vi "SelectFitRange (SubVI).vi"(7 "Fit type":T1, 9 "delta y values":dbl[](array[numeric]), 10 "y values":dbl[](array[numeric]), 11 "x values":dbl[](array[numeric])) -> (1 "Selected delta y values":dbl[](array[numeric]), 2 "Selected y values":dbl[](array[numeric]), 3 "Selected x values":dbl[](array[numeric]))   [LabVIEW 2016]
uses:
  Utils/Enum_TypeDefinitions/Enum_TypeDef_ParabolaFitType.ctl
panel:
  out "Index of extreme":i32
  out "Righthand side":i32
  out "Lefthand side":i32
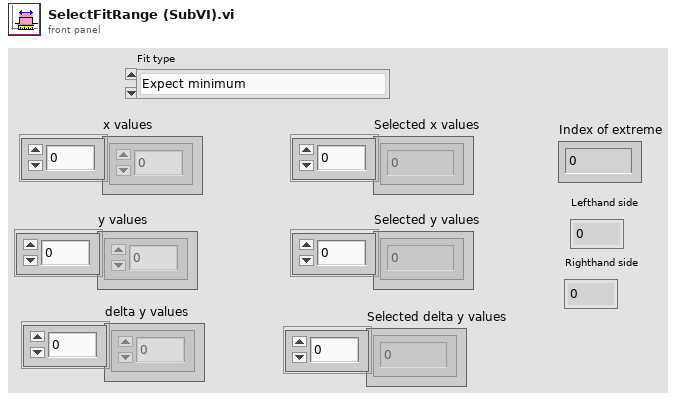
[diagram p1: front panel]
types:
  T1 = typedef "Enum_TypeDef_ParabolaFitType.ctl" = enum16{"Expect minimum", "Expect maximum"}
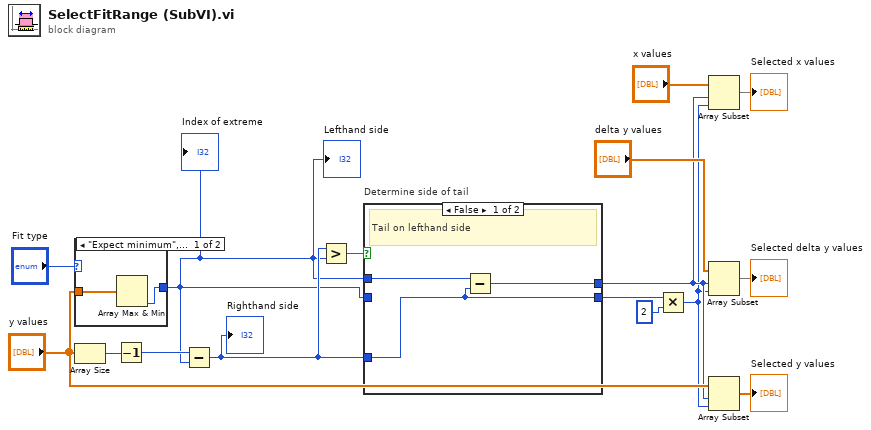
[diagram p0: block diagram]
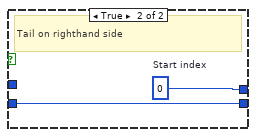
[diagram p2: hidden frame]
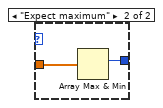
[diagram p3: hidden frame]
diagram:
  n1 = case shown="\"Expect minimum\", Default" "Fit type" {
    tunnel: [w17 w20] -> w5
    tunnel: "y values" -> [w18 w19]
    frame "Expect minimum", Default {
      n2 = Array Max & Min(array=w18) -> (min index (indices)=w17:i32)  [unwired: 3 out]
    }
    frame "Expect maximum" {
      n3 = Array Max & Min(array=w19) -> (max index (indices)=w20:i32)  [unwired: 3 out]
    }
  }
  "Lefthand side" <- w5
  "Index of extreme" <- w5
  n4 = Array Size(array="y values") -> (size(s)=w10:i32)
  n5 = Decrement(x=w10) -> (x-1=w11:i32)
  n6 = Subtract(x=w11, y=w5) -> (x-y=w6:i32)
  "Righthand side" <- w6
  n7 = Greater?(x=w6, y=w5) -> (0:w7:bool)
  n8 = case "Determine side of tail" shown="False" w7 {
    tunnel: [w22 w25] -> w4
    tunnel: w5 -> [_ w25]
    tunnel: w6 -> [w22 _]
    tunnel: w5 -> [w23 _]
    tunnel: [w21 w24] -> w2
    frame False {
      # "Tail on lefthand side"
      n9 = Subtract(x=w23, y=w22) -> (x-y=w21:i32)
    }
    frame True {
      w24 = 0  # Start index
      # "Tail on righthand side"
    }
  }
  n10 = Multiply(x=w4, y=2) -> (x*y=w1:i32)
  n11 = Array Subset(array="x values", index=w2, length=w1) -> (→"Selected x values":dbl[])
  n12 = Array Subset(array="delta y values", index=w2, length=w1) -> (→"Selected delta y values":dbl[])
  n13 = Array Subset(array="y values", index=w2, length=w1) -> (→"Selected y values":dbl[])
